vi "Actor Core.vi"(8 "error in":errorcluster, 11 "WS Test Client in":refnum<class "WS Test Client Subscriber.lvclass">) -> (0 "error out":errorcluster, 3 "Actor out":refnum<class "Actor.lvclass">)   [LabVIEW 2021, in "Secure Echo Broadcast Test With Server Manager.lvlib" / "WS Test Client Subscriber.lvclass"]
doc: "(<B>Filename</B>: Actor Framework.lvlib:Actor.lvclass:Actor Core.vi)\n\nReceives messages to the actor, reacts to them, and initiates any error handling that may shut the actor down.\n\nDescendant classes may override this VI to append parallel tasks for the actor to complete while it handles messages. Overrides use the Call Parent Method node."
uses:
  WS Test Client Subscriber.lvclass
  C:/Program Files/National Instruments/LabVIEW 2021/vi.lib/ActorFramework/Actor/Actor.lvclass
  <vilib>/ActorFramework/Actor/Actor.lvclass
  <vilib>/ActorFramework/Message Enqueuer/Message Enqueuer.lvclass
  WebSocket Actor/WebSocket Client/WebSocket Client.lvclass
  C:/Projects/WebSocket-Actor/WebSocket Actor/WebSocket Connection/WebSocket Connection.lvclass
  WS Test Client Subscriber Messages/Client Connection Handler Msg/Client Connection Handler Msg.lvclass
  C:/Projects/WebSocket-Actor/WebSocket Actor/Abstract Messages/WebSocket Connection Handler Msg/WebSocket Connection Handler Msg.lvclass
  <vilib>/ActorFramework/Actor/Actor.lvclass/Actor.ctl
  <vilib>/ActorFramework/Message Enqueuer/Message Enqueuer.lvclass/Message Enqueuer.ctl
  WS Test Client Subscriber.lvclass/WS Test Client Subscriber.ctl
  WebSocket Actor/WebSocket Connection/WebSocket Connection.lvclass/WebSocket Connection.ctl
  WebSocket Actor/WebSocket Client/WebSocket Client.lvclass/WebSocket Client.ctl
  WebSocket Actor/WebSocket Connection/properties/Write Timeout.vi
  WebSocket Actor/WebSocket Connection/properties/Write WebSocket Data Handler.vi
  WebSocket Actor/WebSocket Connection/Write Keepalive.vi
  WebSocket Actor/WebSocket Client/Write Certificate.vi
  <vilib>/ActorFramework/Message Enqueuer/Init from Existing Queue.vi
  WebSocket Actor/WebSocket Client/properties/Write WS URI.vi
  WebSocket Actor/WebSocket Connection Messages/Send to Peer Msg/Send to Peer Msg.lvclass
  <userlib>/_OpenG.lib/time/time.llb/openg_time.lvlib
  <userlib>/_OpenG.lib/error/error.llb/openg_error.lvlib
panel:
  in  "Send":bool
  in  "Data To Send":string
  out "Echoed Data":string
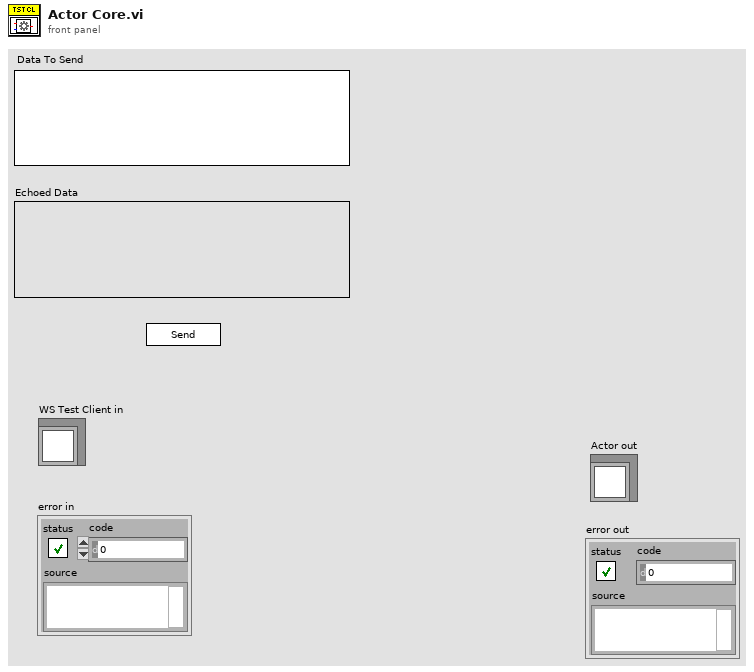
[diagram p1: front panel]
types:
  T1 = typedef "WebSocket Actors.lvlib/WebSocket Connection.lvclass/Keepalive.ctl" = cluster{"Enabled":bool, "Ping Interval (ms)":u32, "Ping Timeout (ms)":u32}
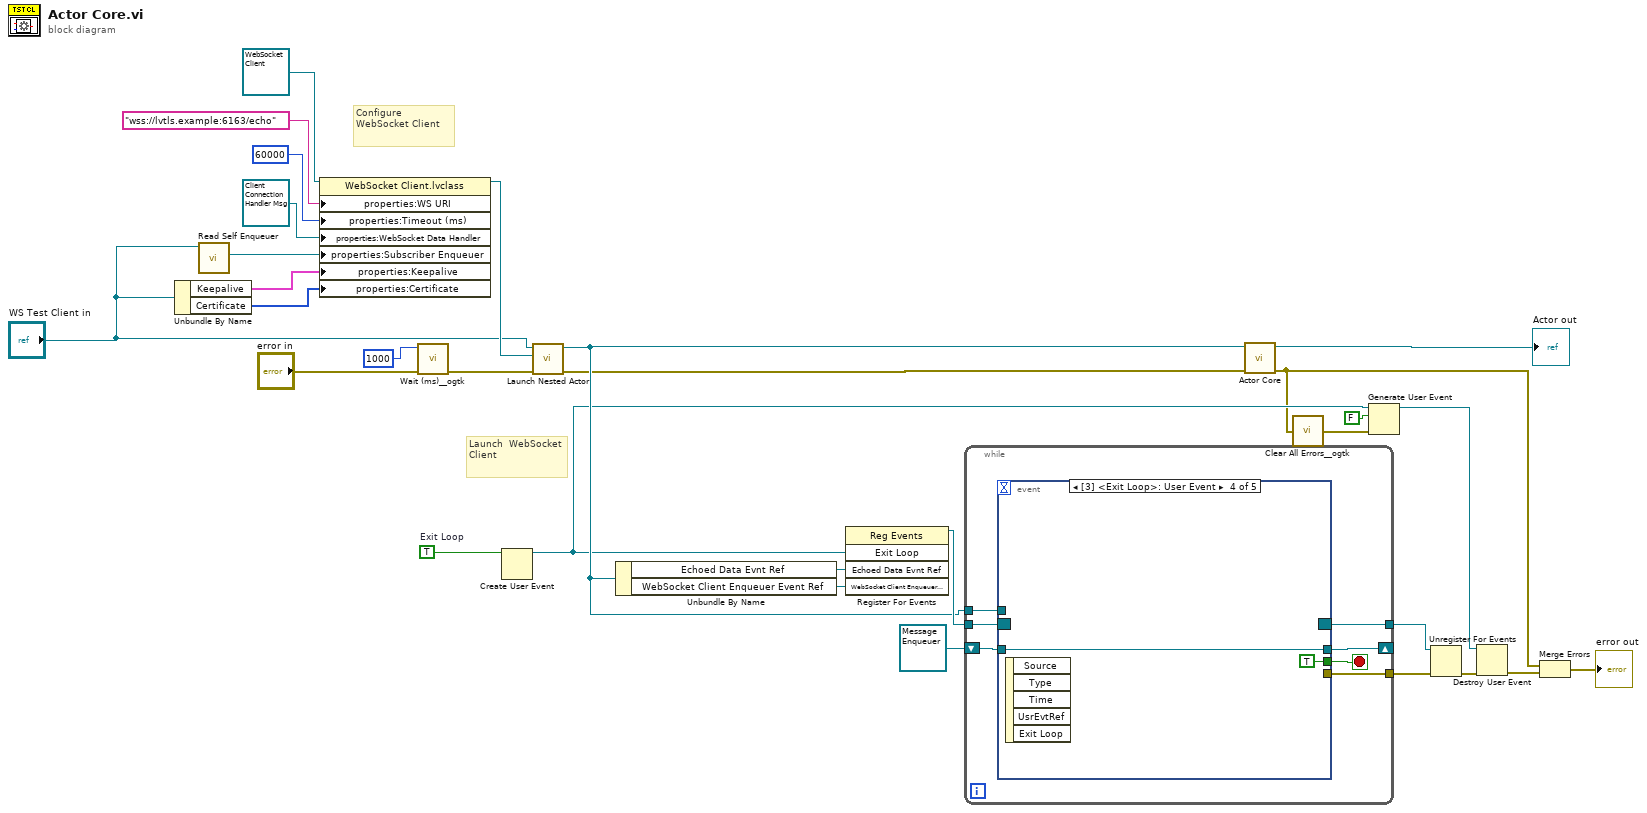
[diagram p0: block diagram]
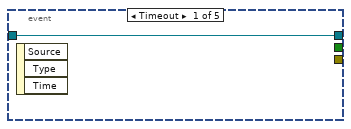
[diagram p2: hidden frame]
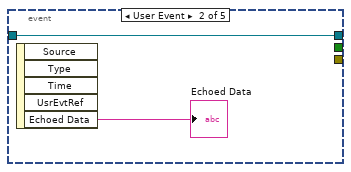
[diagram p3: hidden frame]
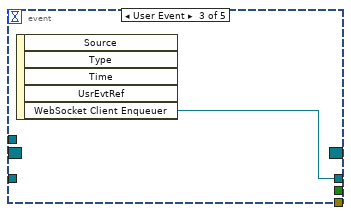
[diagram p4: hidden frame]
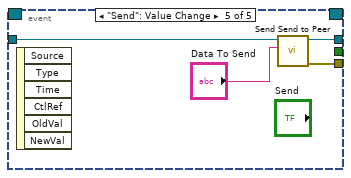
[diagram p5: hidden frame]
diagram:
  w12 = TRUE  # Exit Loop
  # "Configure  WebSocket Client"
  # "Launch  WebSocket Client"
  n1 = Unbundle By Name("WS Test Client in") -> ("Keepalive"=w2:T1, "Certificate"=w1:u8[])
  n2 = call <vilib>:"Read Self Enqueuer.vi"("Actor"="WS Test Client in") -> ("Self Enqueuer"=w15:refnum<class "Message Enqueuer.lvclass">)  [unwired: 10 in]
  n3 = property class="WebSocket Client.lvclass"(reference=refnum<class "WebSocket Client.lvclass"> refnum ("WebSocket Actors.lvlib:WebSocket Client.lvclass"), "properties:WS URI"="wss://lvtls.example:6163/echo" ("Address"), "properties:Timeout (ms)"=60000 ("Timeout (60000 ms)"), "properties:WebSocket Data Handler"=refnum<class "Client Connection Handler Msg.lvclass"> refnum ("WS Full LabVIEW Test.lvlib:Client Connection Handler Msg.lvclass"), "properties:Subscriber Enqueuer"=w15, "properties:Keepalive"=w2, "properties:Certificate"=w1) -> (reference out=w20:refnum<class "WebSocket Client.lvclass">)  [unwired: 1 in, 1 out]
  n4 = call <userlib>:"Wait (ms)__ogtk.vi"("error in (no error)"="error in", "milliseconds to wait"=u32 1000) -> ("error out"=w17:errorcluster)  [unwired: 8 in, 1 out]
  n5 = Create User Event(user event datatype=w12) -> (user event=w9:refnum<user-event>)  [unwired: 1 in, 1 out]
  n6 = call <vilib>:"Launch Nested Actor.vi"("error in (no error)"=w17, "Nested Actor"=w20, "Caller Actor in"="WS Test Client in") -> ("error out"=w11:errorcluster, "Caller Actor out"=w13:refnum<class "WS Test Client Subscriber.lvclass">)  [unwired: 6 in, 1 out]
  n7 = Unbundle By Name(w13) -> ("Echoed Data Evnt Ref"=w29:refnum<user-event>, "WebSocket Client Enqueuer Event Ref"=w27:refnum<user-event>)
  n8 = register-events(w9, w29, w27) -> (reference out=w28:refnum<event-registration>)  [unwired: 2 in, 1 out]
  n9 = while {
    tunnel: w28 -> [w37]
    shift-right: [w35] -> _
    shift-left: refnum<class "Message Enqueuer.lvclass"> refnum ("WebSocket Client Enqueuer") -> [w34]
    tunnel: [w33] -> w25
    tunnel: w13 -> [w32]
    tunnel: [w31] -> w23
    stop <- w36 stop-if-true
    n10 = event shown="[3] <Exit Loop>: User Event" {
      selector: w37 -> [_ _ _ _ _]
      dyn-events: [_ _ _ _ _] -> w33
      timeout: _ -> [_ _ _ _ _]
      tunnel: [_ _ _ TRUE ("Exit") _] -> w36
      tunnel: [w38 w39 w41 w43 w45] -> w35
      tunnel: w34 -> [w38 w39 _ w43 w46]
      tunnel: w32 -> [_ _ _ _ _]
      tunnel: [_ _ _ _ w44] -> w31
      event Timeout {
        n11 = event-data() -> ()  [unwired: 1 in, 3 out]
      }
      event User Event {
        n12 = event-data() -> ("Echoed Data"=→"Echoed Data":string)  [unwired: 1 in, 4 out]
      }
      event User Event {
        n13 = event-data() -> ("WebSocket Client Enqueuer"=w41:refnum<class "Message Enqueuer.lvclass">)  [unwired: 1 in, 4 out]
      }
      event User Event {
        n14 = event-data() -> ()  [unwired: 1 in, 5 out]
      }
      event "Send": Value Change {
        n15 = event-data() -> ()  [unwired: 1 in, 6 out]
        n16 = call "Send Send to Peer.vi"("Data"="Data To Send", "Message Enqueuer in"=w46) -> ("error out"=w44:errorcluster, "Message Enqueuer out"=w45:refnum<class "Message Enqueuer.lvclass">)  [unwired: 8 in]
      }
    }
  }
  n17 = call-parent "Actor Core.vi"("error in"=w11, "Actor in"=w13) -> ("error out"=w4:errorcluster, "Actor out"=→"Actor out":refnum<class "Actor.lvclass">)  [unwired: 8 in]
  n18 = call <userlib>:"Clear All Errors__ogtk.vi"("Error In"=w4) -> ("Error Out"=w10:errorcluster)  [unwired: 3 in]
  n19 = Generate User Event(user event=w9, event data cluster=FALSE ("event data"), error in=w10) -> (user event out=w7:refnum<user-event>)  [unwired: 1 in, 1 out]
  n20 = Unregister For Events(event registration refnum=w25, error in=w23) -> (error out=w6:errorcluster)
  n21 = Destroy User Event(user event=w7, error in=w6) -> (error out=w5:errorcluster)
  n22 = Merge Errors(w4, w5) -> (→"error out":errorcluster)
